vi "Init Device.vi"(8 "error in (no error)":errorcluster, 11 "Orca-Flash 4.0 in":refnum<class "Orca-Flash 4.0 V2.lvclass">) -> (0 "error out":errorcluster, 3 "Orca-Flash 4.0 out":refnum<class "Orca-Flash 4.0 V2.lvclass">)   [LabVIEW 2018, in "Orca-Flash 4.0 V2.lvlib" / "Orca-Flash 4.0 V2.lvclass"]
uses:
  Orca-Flash 4.0 V2.lvclass
  C:/FlashGordon/Hardware/Camera/Camera.lvclass
  Resources/Type Defs/Physical Camera Assignment.ctl
  Resources/Type Defs/Camera Type.ctl
  Orca-Flash 4.0 V2.lvclass/Orca-Flash 4.0 V2.ctl
  Resources/GLOBAL/GLOBAL Time-critical.vi
  Camera/Camera.lvclass
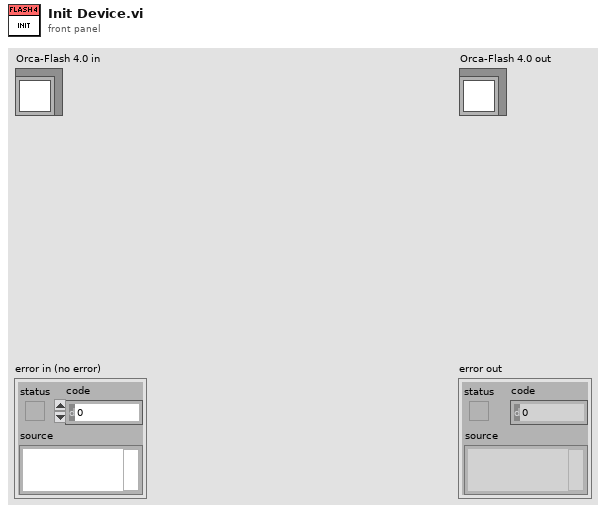
[diagram p1: front panel]
types:
  T1 = typedef "Physical Camera Assignment.ctl" = cluster{"Channel Name":string, "Camera Type":T2, "Serial Number":string, "Flip Vertically":bool, "Flip Horizontally":bool, "photonsPerCount":dbl, "wavelength":i16}
  T2 = typedef "Camera Type.ctl" = enum16{"Hamamatsu"}
  T3 = cluster{"Model":string, "Camera ID":string, "Firmware":string}[]
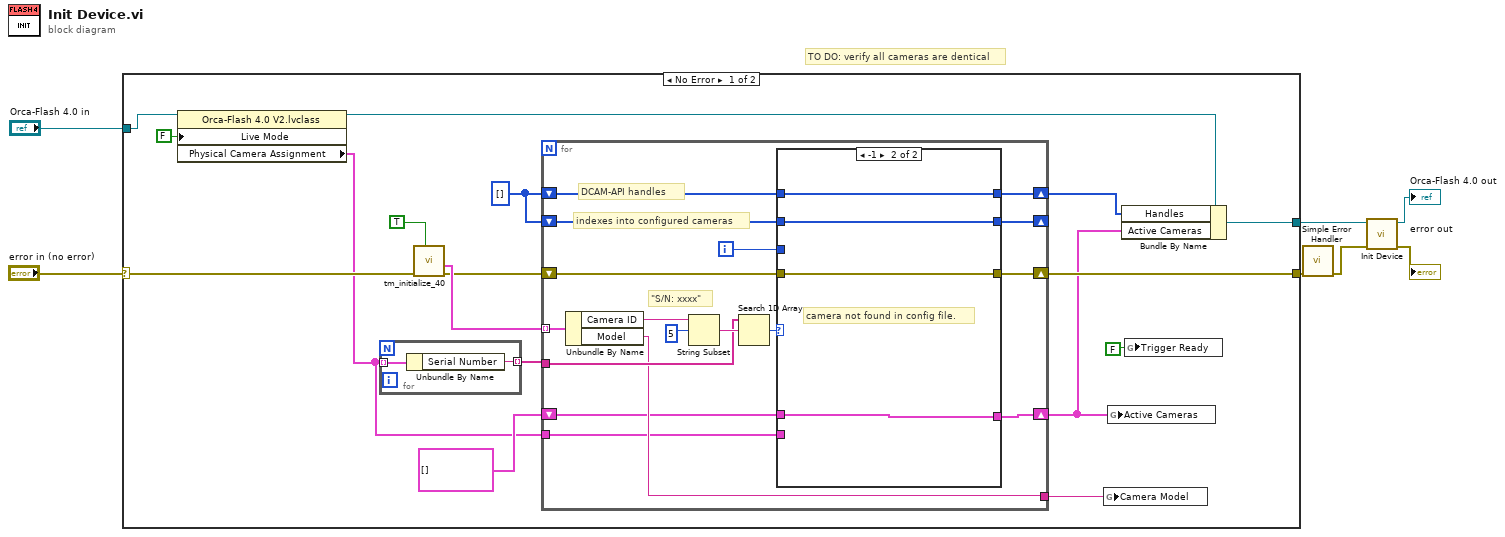
[diagram p0: block diagram]
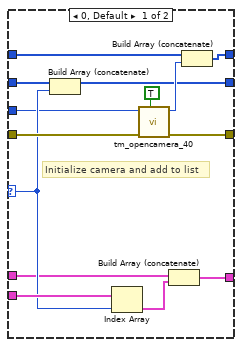
[diagram p2: hidden frame]
diagram:
  # "TO DO: verify all cameras are dentical"
  n1 = case shown="No Error" "error in (no error)" {
    selector: "error in (no error)" -> [w24 w63]
    tunnel: [w18 w63] -> w2
    tunnel: "Orca-Flash 4.0 in" -> [w15 w62]
    tunnel: [w23 w62] -> w3
    frame No Error {
      w19 = u32[] []
      n2 = property class="Orca-Flash 4.0 V2.lvclass"(reference=w15, "Live Mode"=FALSE) -> (reference out=w14:refnum<class "Orca-Flash 4.0 V2.lvclass">, "Physical Camera Assignment"=w10:T1[])  [unwired: 1 in, 1 out]
      n3 = for {
        tunnel: w10 -> [w61] mode=indexing
        tunnel: [w60] -> w21 mode=indexing
        n4 = Unbundle By Name(w61) -> ("Serial Number"=w60:string)
      }
      n5 = call <userlib>:"tm_initialize_40.vi"("HVCC Log (F)"=TRUE, "error in (no error)"=w24) -> ("error out"=w20:errorcluster, "Camera Details Array"=w22:T3)  [unwired: 6 in, 2 out]
      n6 = for {
        tunnel: w22 -> [w41] mode=indexing
        tunnel: w21 -> [w37]
        shift-right: [w34] -> w18
        shift-left: w20 -> [w35]
        shift-right: [w33] -> w16
        shift-left: w19 -> [w30]
        shift-right: [w31] -> _
        shift-left: w19 -> [w32]
        tunnel: [w29] -> w17
        tunnel: w10 -> [w27]
        shift-right: [w28] -> w9
        shift-left: T1[] [] -> [w26]
        i -> [w25]
        # "indexes into configured cameras"
        # "DCAM-API handles"
        # "\"S/N: xxxx\""
        n7 = Unbundle By Name(w41) -> ("Camera ID"=w40:string, "Model"=w29:string)
        n8 = String Subset(string=w40, offset (0)=5) -> (substring=w38:string)  [unwired: 1 in]
        n9 = Search 1D Array(1D array=w37, element=w38) -> (index of element=w36:i32)  [unwired: 1 in]
        n10 = case shown="-1" w36 {
          selector: w36 -> [w46 _]
          tunnel: w35 -> [w55 w59]
          tunnel: [w54 w59] -> w34
          tunnel: w30 -> [w50 w58]
          tunnel: [w51 w58] -> w33
          tunnel: w32 -> [w48 w57]
          tunnel: [w47 w57] -> w31
          tunnel: [w45 w56] -> w28
          tunnel: w27 -> [w52 _]
          tunnel: w26 -> [w43 w56]
          tunnel: w25 -> [w42 _]
          frame 0, Default {
            # "Initialize camera and add to list"
            n11 = Build Array (concatenate)(w48, w46) -> (w47:u32[])
            n12 = Index Array(array=w52, index=w46) -> (element=w44:T1)
            n13 = call <userlib>:"tm_opencamera_40.vi"("Force Open"=TRUE, "error in (no error)"=w55, "Camera Index"=w42) -> ("error out"=w54:errorcluster, "Handle out"=w49:u32)  [unwired: 6 in, 1 out]
            n14 = Build Array (concatenate)(w43, w44) -> (w45:T1[])
            n15 = Build Array (concatenate)(w50, w49) -> (w51:u32[])
          }
          frame -1 {
            # "camera not found in config file."
          }
        }
      }
      n16 = global write "GLOBAL Time-critical.vi" "Camera Model"(w17) -> ()
      n17 = global write "GLOBAL Time-critical.vi" "Active Cameras"(w9) -> ()
      n18 = Bundle By Name(cluster=w14, "Handles"=w16, "Active Cameras"=w9) -> (w23:refnum<class "Orca-Flash 4.0 V2.lvclass">)
      n19 = global write "GLOBAL Time-critical.vi" "Trigger Ready"(FALSE) -> ()
    }
    frame Error {
    }
  }
  n20 = call <vilib>:"Simple Error Handler.vi"("error in (no error)"=w2) -> ("error out"=w1:errorcluster)  [unwired: 4 in, 4 out]
  n21 = call-parent "Init Device.vi"("error in (no error)"=w1, "Camera in"=w3) -> ("error out"=→"error out":errorcluster, "Camera out"=→"Orca-Flash 4.0 out":refnum<class "Orca-Flash 4.0 V2.lvclass">)  [unwired: 8 in]
